vi "read.vi"(8 "error in (no error)":errorcluster, 10 "ILC":refnum<class "ILC.lvclass">, 11 "IReadILCStrategy in":refnum<class "IReadILCStrategy.lvclass">) -> (0 "error out":errorcluster, 2 "Value":dbl, 3 "IReadILCStrategy out":refnum<class "IReadILCStrategy.lvclass">)   [LabVIEW 2015, in "IReadILCStrategy.lvclass"]
uses:
  IReadILCStrategy.lvclass
  <userlib>/Common/ILC/ILC/ILC.lvclass
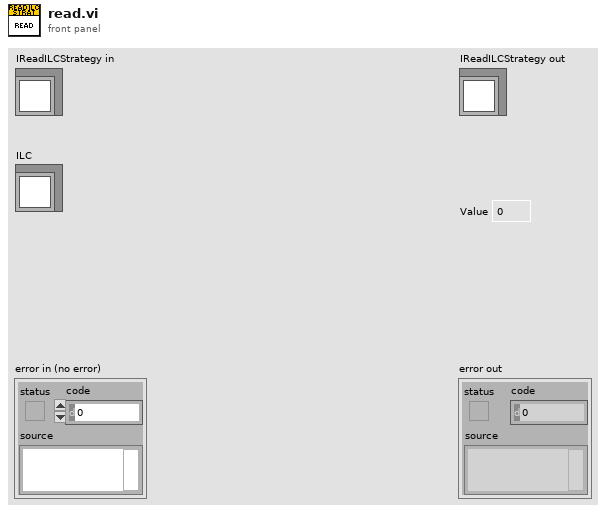
[diagram p1: front panel]
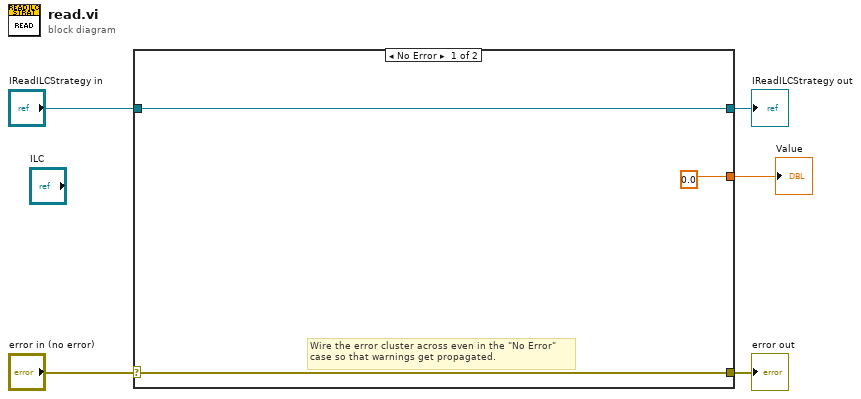
[diagram p0: block diagram]
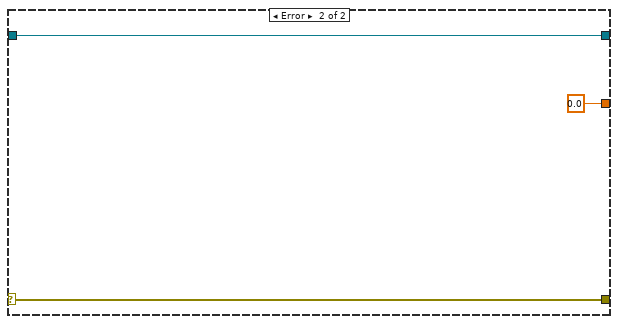
[diagram p2: hidden frame]
diagram:
  n1 = case shown="No Error" "error in (no error)" {
    selector: "error in (no error)" -> [w7 w11]
    tunnel: [w7 w11] -> w4
    tunnel: [w8 w10] -> w2
    tunnel: "IReadILCStrategy in" -> [w8 w10]
    tunnel: [0.0 ("Value") 0.0 ("Value")] -> w1
    frame No Error {
      # "Wire the error cluster across even in the \"No Error\"\ncase so that warnings get propagated."
    }
    frame Error {
    }
  }
  "error out" <- w4
  "IReadILCStrategy out" <- w2
  "Value" <- w1
